vi "Select or Unselect GU.vi"(6 "Add/Del(T:Add)":bool=TRUE, 8 "error in":errorcluster, 10 "Curr Cal Cfg":T1, 11 "GU List":refnum<vi>) -> (0 "error out":errorcluster, 2 "Curr Cal Cfg Out":T1)   [LabVIEW 2020, in "GUCalibration2.lvlib"]
uses:
  GUCalibration2.lvlib
  Controls/Config Data Type.ctl
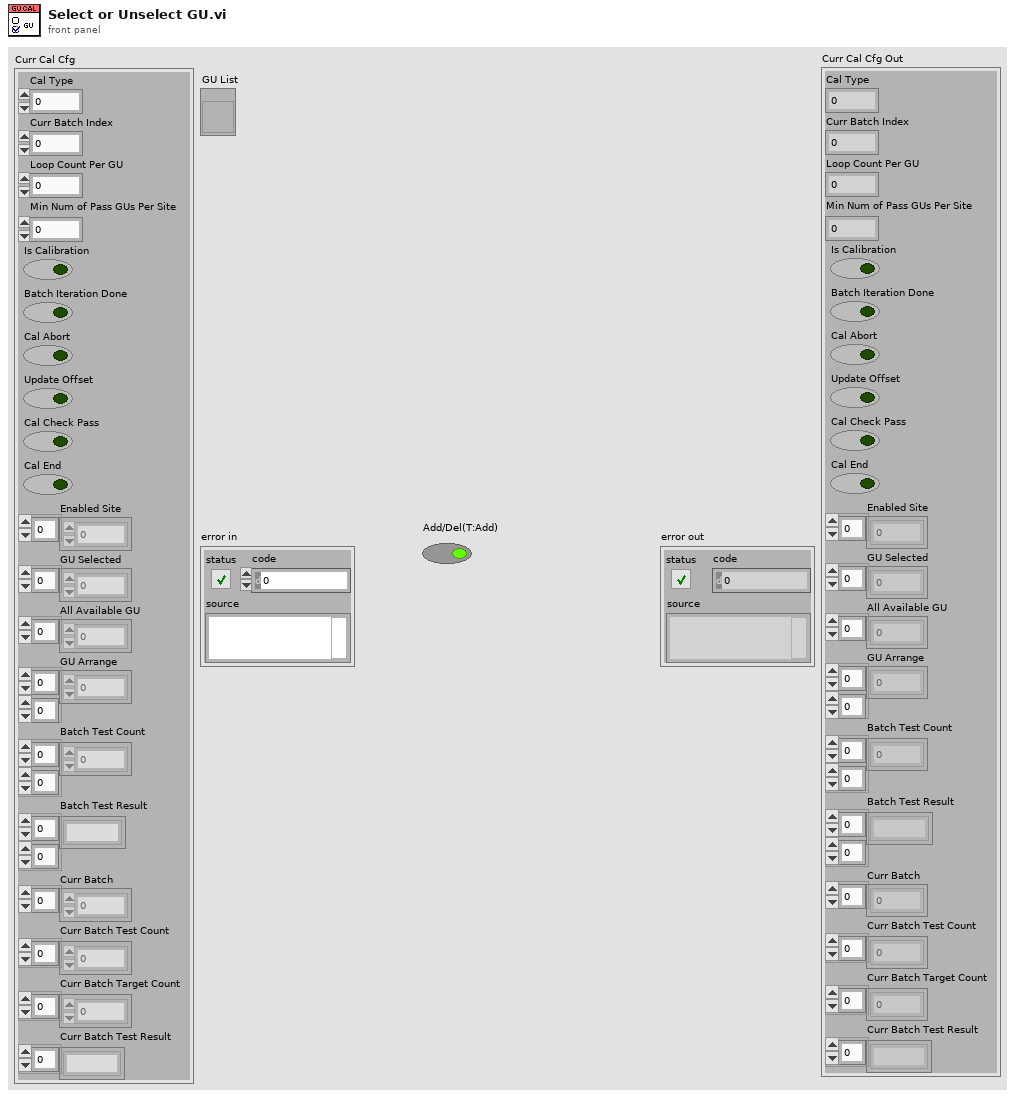
[diagram p1: front panel]
types:
  T1 = typedef "GUCalibration2.lvlib/Config Data Type.ctl" = cluster{"Cal Type":i32, "Curr Batch Index":i32, "Loop Count Per GU":i32, "Min Num of Pass GUs Per Site":i32, "Is Calibration":bool, "Batch Iteration Done":bool, "Cal Abort":bool, "Update Offset":bool, "Cal Check Pass":bool, "Cal End":bool, "Enabled Site":i32[], "GU Selected":i32[], "All Available GU":i32[], "GU Arrange":i32[][], "Batch Test Count":i32[][], "Batch Test Result":string[][], "Curr Batch":i32[], "Curr Batch Test Count":i32[], "Curr Batch Target Count":i32[], "Curr Batch Test Result":string[]}
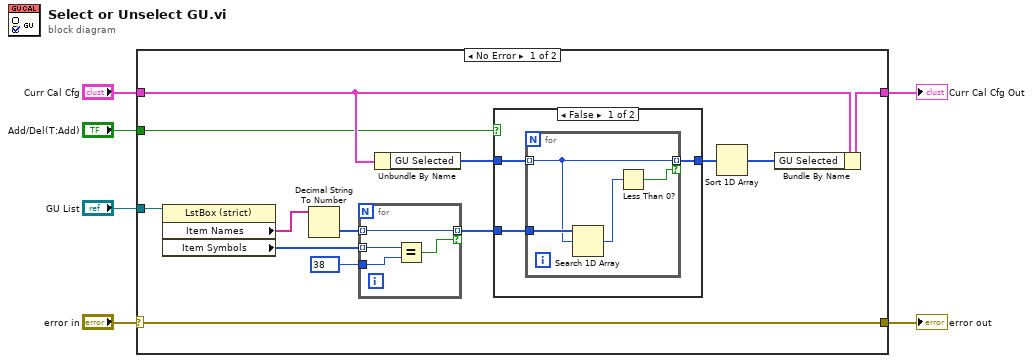
[diagram p0: block diagram]
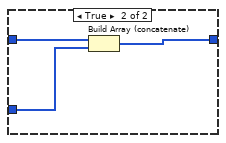
[diagram p2: hidden frame]
diagram:
  n1 = case shown="No Error" "error in" {
    selector: "error in" -> [w7 w34]
    tunnel: "GU List" -> [w18 _]
    tunnel: "Curr Cal Cfg" -> [w11 w35]
    tunnel: [w9 w35] -> w4
    tunnel: "Add/Del(T:Add)" -> [w8 _]
    tunnel: [w7 w34] -> w1
    frame No Error {
      n2 = property class="LstBox (strict)"(reference=w18) -> ("Item Names"=w16:string[], "Item Symbols"=w19:i32[])  [unwired: 1 in, 2 out]
      n3 = Decimal String To Number(string=w16) -> (number=w15:i32[])  [unwired: 2 in, 1 out]
      n4 = for {
        tunnel: w15 -> [w31] mode=indexing
        tunnel: w19 -> [w33] mode=indexing
        tunnel: 38 -> [w32]
        tunnel: [w31] -> w13 mode=indexing if=w30
        n5 = Equal?(x=w33, y=w32) -> (x = y?=w30:bool)
      }
      n6 = Unbundle By Name(w11) -> ("GU Selected"=w14:i32[])
      n7 = case shown="False" w8 {
        tunnel: w14 -> [w22 w29]
        tunnel: w13 -> [w21 w28]
        tunnel: [w20 w27] -> w12
        frame False {
          n8 = for {
            tunnel: w22 -> [w24] mode=indexing
            tunnel: w21 -> [w26]
            tunnel: [w24] -> w20 mode=indexing if=w23
            n9 = Search 1D Array(1D array=w26, element=w24) -> (index of element=w25:i32)  [unwired: 1 in]
            n10 = Less Than 0?(x=w25) -> (x < 0?=w23:bool)
          }
        }
        frame True {
          n11 = Build Array (concatenate)(w29, w28) -> (w27:i32[])
        }
      }
      n12 = Sort 1D Array(array=w12) -> (sorted array=w10:i32[])
      n13 = Bundle By Name(cluster=w11, "GU Selected"=w10) -> (w9:T1)
    }
    frame Error {
    }
  }
  "Curr Cal Cfg Out" <- w4
  "error out" <- w1
